vi "Progress Bar.vi"() -> ()   [LabVIEW 2015]
uses:
  Progress Bar Cluster.ctl
  Progress Bar Action.ctl
panel:
  out "State":string
  out "progress":u32(slide) scale=0.0..100.0
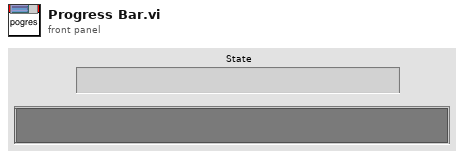
[diagram p1: front panel]
types:
  T1 = typedef "Progress Bar Cluster.ctl" = cluster{"Action":T2, "State":string, "Progress (0-1)":dbl}
  T2 = typedef "Progress Bar Action.ctl" = enum16{"Open", "Update", "Close", "End"}
  T3 = enum32{"Invalid", "Standard", "Closed", "Hidden", "Minimized", "Maximized"}
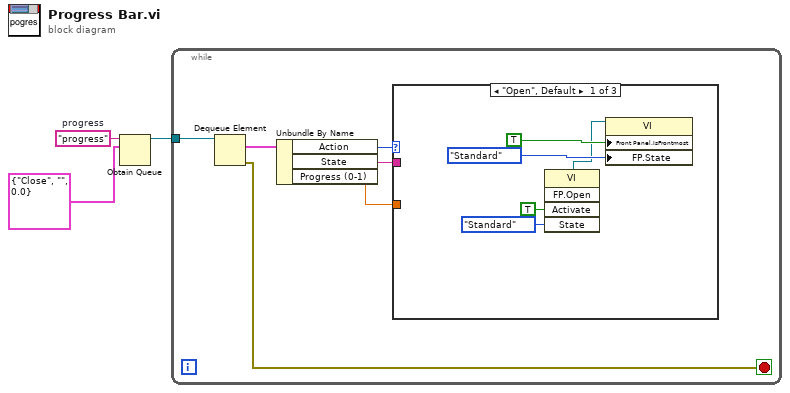
[diagram p0: block diagram]
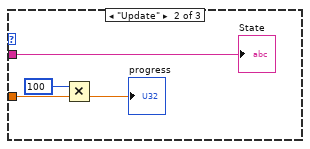
[diagram p2: hidden frame]
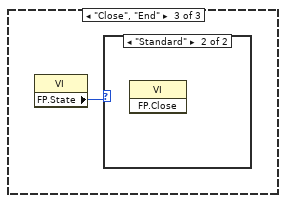
[diagram p3: hidden frame]
diagram:
  w3 = "progress"  # progress
  n1 = Obtain Queue(name (unnamed)=w3, element data type=T1 {"Action"=enum."Close", "State"="", "Progress (0-1)"=0.0}) -> (queue out=w1:refnum<queue>)  [unwired: 3 in, 2 out]
  n2 = while {
    tunnel: w1 -> [w9]
    stop <- w8 stop-if-true
    n3 = Dequeue Element(queue=w9) -> (element=w7:T1, error out=w8:errorcluster)  [unwired: 2 in, 2 out]
    n4 = Unbundle By Name(w7) -> ("Action"=w6:T2, "State"=w5:string, "Progress (0-1)"=w4:dbl)
    n5 = case shown="\"Open\", Default" w6 {
      tunnel: w5 -> [_ w18 _]
      tunnel: w4 -> [_ w17 _]
      frame "Open", Default {
        n6 = invoke class="VI" method="FP.Open"("Activate"=TRUE ("Activate?"), "State"=T3."Standard") -> (reference out=w10:refnum<vi>)  [unwired: 3 in, 4 out]
        n7 = property class="VI"(reference=w10, "Front Panel.IsFrontmost"=TRUE ("Front Panel Window:Is Frontmost"), "FP.State"=T3."Standard" ("Front Panel Window:State")) -> ()  [unwired: 1 in, 2 out]
      }
      frame "Update" {
        n8 = Multiply(x=100, y=w17) -> (x*y=→"progress":dbl)
        "State" <- w18
      }
      frame "Close", "End" {
        n9 = property class="VI"() -> ("FP.State"=w19:T3)  [unwired: 2 in, 2 out]
        n10 = case shown="\"Standard\"" w19 {
          frame "Invalid", Default {
          }
          frame "Standard" {
            n11 = invoke class="VI" method="FP.Close"() -> ()  [unwired: 3 in, 3 out]
          }
        }
      }
    }
  }
